vi "MultiplyArray.vi"(6 "Calibration":sgl, 9 "DataIn":sgl[][](array[numeric]), 10 "Pixels/Line":u16, 11 "Lines":i32) -> (1 "MultipliedData":sgl[][](array[numeric]))   [LabVIEW 2016]
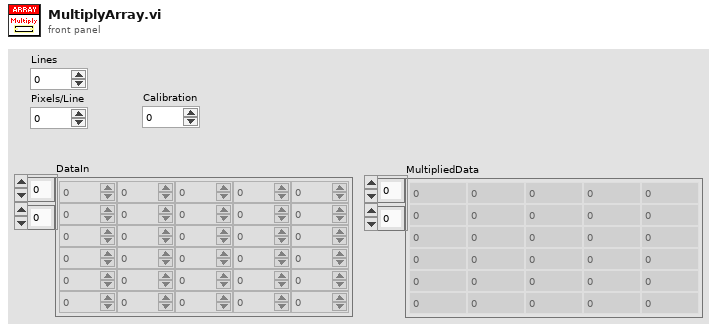
[diagram p1: front panel]
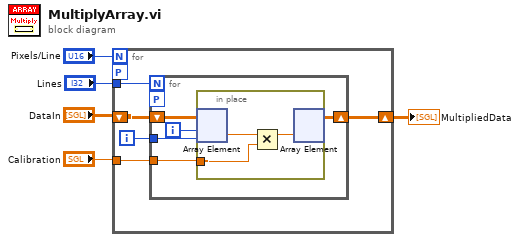
[diagram p0: block diagram]
diagram:
  n1 = for {
    N: "Pixels/Line" -> [_]
    tunnel: "Calibration" -> [w10]
    tunnel: "Lines" -> [w7]
    shift-right: [w9] -> w3
    shift-left: "DataIn" -> [w8]
    workers-P: _ -> [_]
    i -> [w6]
    n2 = for {
      N: w7 -> [_]
      tunnel: w10 -> [w14]
      tunnel: w6 -> [w11]
      shift-right: [w13] -> w9
      shift-left: w8 -> [w15]
      workers-P: _ -> [_]
      i -> [w12]
      n3 = in-place {
        in-place-border: w14 -> [w17]
        n4 = in-place-array #1(w15, w12, w11) -> (w18:sgl)
        n5 = Multiply(x=w18, y=w17) -> (x*y=w16:sgl)
        n6 = in-place-array #1(w16) -> (w13:sgl[][])  [unwired: 2 out]
      }
    }
  }
  "MultipliedData" <- w3
